vi "Parse.vi"(8 "error in (no error)":errorcluster, 11 "Transform.Skew in":refnum<class "Transform.Skew.lvclass">) -> (0 "error out":errorcluster, 3 "Transform.Skew out":refnum<class "Transform.Skew.lvclass">)   [LabVIEW 2019, in "Transform.Skew.lvclass"]
uses:
  Transform.Skew.lvclass
  C:/Users/Albro/Documents/GitHub/AFM-Lithography/lvsrc/Classes/Parse/Transform/Transform.lvclass
  Transform/Transform.lvclass/Transform.ctl
  Transform/Transform.lvclass
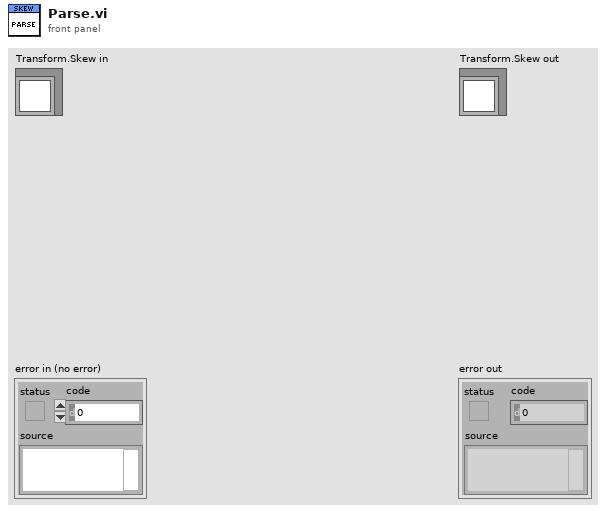
[diagram p1: front panel]
types:
  T1 = typedef "NI_Matrix.lvlib/RealMatrix.ctl" = dbl[][]
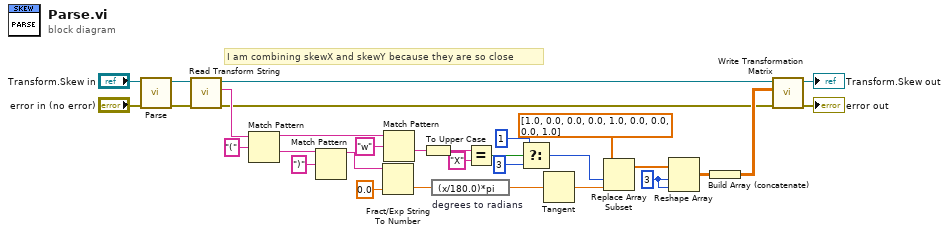
[diagram p0: block diagram]
diagram:
  w7 = 3 ("dimension size")
  # "I am combining skewX and skewY because they are so close"
  n1 = call-parent "Parse.vi"("error in (no error)"="error in (no error)", "Transform in"="Transform.Skew in") -> ("error out"=w3:errorcluster, "Transform out"=w29:refnum<class "Transform.Skew.lvclass">)  [unwired: 8 in]
  n2 = call "Read Transform String.vi"("error in (no error)"=w3, "Transform in"=w29) -> ("error out"=w4:errorcluster, "Transform String"=w26:string, "Transform out"=w28:refnum<class "Transform.Skew.lvclass">)  [unwired: 7 in]
  n3 = Match Pattern(string=w26, regular expression="(") -> (before substring=w21:string, after substring=w24:string)  [unwired: 1 in, 2 out]
  n4 = Match Pattern(string=w24, regular expression=")") -> (before substring=w1:string)  [unwired: 1 in, 3 out]
  n5 = Fract/Exp String To Number(string=w1, default (0 dbl)=0.0 ("default (0 DBL)")) -> (number=w11:dbl)  [unwired: 2 in, 1 out]
  n6 = Match Pattern(string=w21, regular expression="w") -> (after substring=w20:string)  [unwired: 1 in, 3 out]
  n7 = To Upper Case(1:w20) -> (0:w19:string)
  n8 = expression code="(x/180.0)*pi" "degrees to radians"(w11) -> (w10:dbl)
  n9 = Equal?(x=w19, y="X") -> (x = y?=w18:bool)
  n10 = Select(t=1, s=w18, f=3) -> (s? t:f=w12:i32)
  n11 = Tangent(1:w10) -> (0:w9:dbl)
  n12 = Replace Array Subset(array=dbl[] [1.0, 0.0, 0.0, 0.0, 1.0, 0.0, 0.0, 0.0, 1.0], new element=w9, index=w12) -> (w8:dbl[])
  n13 = Reshape Array(w8, w7, w7) -> (w6:dbl[][])
  n14 = Build Array (concatenate)(w6) -> (w5:T1)
  n15 = call "Write Transformation Matrix.vi"("error in (no error)"=w4, "Real Matrix"=w5, "Transform in"=w28) -> ("error out"=→"error out":errorcluster, "Transform out"=→"Transform.Skew out":refnum<class "Transform.Skew.lvclass">)  [unwired: 7 in]
